vi "SetCalcData.vi"(8 "error in (no error)":errorcluster caption="entrée d'erreur (pas d'erreur)", 9 "DataQRefs":refnum<queue>[](array[refnum]), 10 "ScanDataQ":string[](array[string]), 11 "Experiment en entrée":refnum<class "Experiment.lvclass"> caption="DNL_LabVIEW Object in") -> (0 "error out":errorcluster caption="sortie d'erreur", 3 "Experiment en sortie":refnum<class "Experiment.lvclass"> caption="DNL_LabVIEW Object out")   [LabVIEW 2019, in "Experiment.lvclass"]
uses:
  Experiment.lvclass
  Experiment.lvclass/Experiment.ctl
  Calculations Class/Calculations.lvclass
  C:/Programmes Labview/LabscanV1A/DevicesClass/BaseDevice/BaseDevice.lvclass
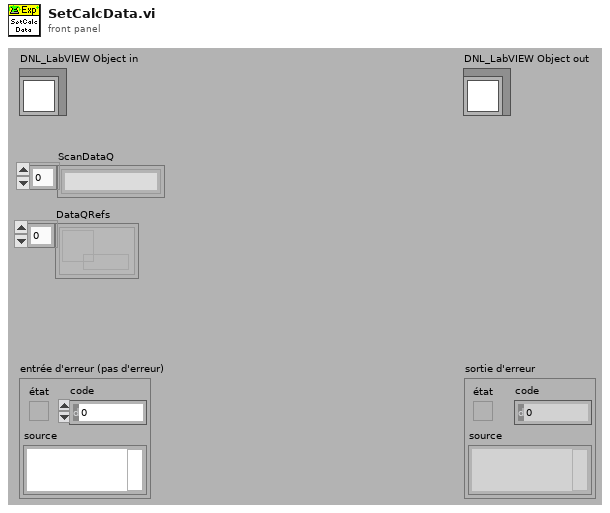
[diagram p1: front panel]
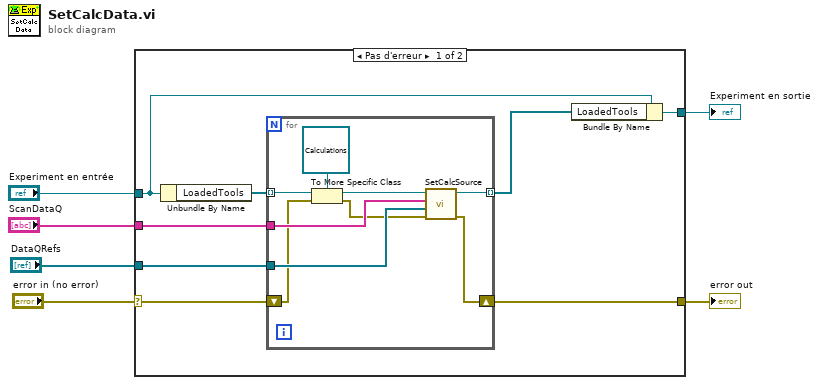
[diagram p0: block diagram]
diagram:
  n1 = case shown="Pas d'erreur" "error in (no error)" {
    selector: "error in (no error)" -> [w11 w25]
    tunnel: [w10 w25] -> w5
    tunnel: [w8 w24] -> w3
    tunnel: "Experiment en entrée" -> [w9 w24]
    tunnel: "ScanDataQ" -> [w12 _]
    tunnel: "DataQRefs" -> [w13 _]
    frame No Error {
      n2 = Unbundle By Name(w9) -> ("LoadedTools"=w14:refnum<class "BaseDevice.lvclass">[])
      n3 = for {
        tunnel: w14 -> [w23] mode=indexing
        tunnel: w13 -> [w19]
        tunnel: w12 -> [w20]
        shift-right: [w18] -> w10
        shift-left: w11 -> [w15]
        tunnel: [w17] -> w7 mode=indexing
        n4 = To More Specific Class(target class=refnum<class "Calculations.lvclass"> refnum ("Calculations.lvclass"), reference=w23, error in=w15) -> (specific class reference=w22:refnum<class "Calculations.lvclass">, error out=w16:errorcluster)
        n5 = call "SetCalcSource.vi"("error in (no error)"=w16, "DataQRefs"=w19, "ScanDataQ"=w20, "InstrClassIn"=w22) -> ("error out"=w18:errorcluster, "InstrClassOut"=w17:refnum<class "Calculations.lvclass">)  [unwired: 6 in]
      }
      n6 = Bundle By Name(cluster=w9, "LoadedTools"=w7) -> (w8:refnum<class "Experiment.lvclass">)
    }
    frame Error {
    }
  }
  "error out" <- w5
  "Experiment en sortie" <- w3
